vi "Set MAX Volts.vi"(8 "error in (no error)":errorcluster, 11 "VISA resource name":refnum<visa-resource-name>) -> (0 "error out":errorcluster, 3 "VISA resource name out":refnum<visa-resource-name>)   [LabVIEW 2010, in "Agilent U2722.lvlib"]
doc: "Configures the channel to output in source voltage mode."
uses:
  U2722 LabVIEW Instr Driver and Examples/Agilent U2722.lvlib
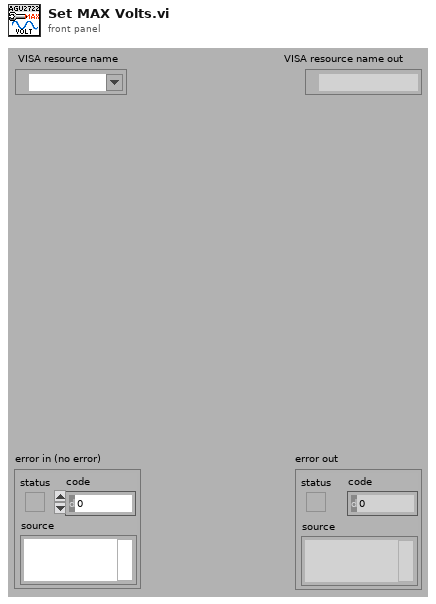
[diagram p1: front panel]
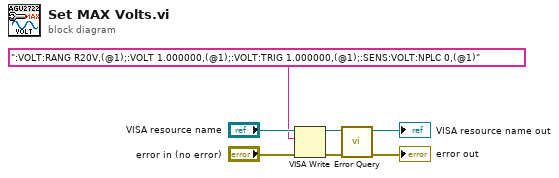
[diagram p0: block diagram]
diagram:
  n1 = VISA Write(VISA resource name="VISA resource name", write buffer=":VOLT:RANG R20V,(@1);:VOLT 1.000000,(@1);:VOLT:TRIG 1.000000,(@1);:SENS:VOLT:NPLC 0,(@1)" ("resulting string"), error in (no error)="error in (no error)") -> (VISA resource name out=w3:refnum<visa-resource-name>, error out=w2:errorcluster)  [unwired: 1 out]
  n2 = call "Error Query.vi"("error in (no error)"=w2, "VISA resource name"=w3) -> ("error out"=→"error out":errorcluster, "VISA resource name out"=→"VISA resource name out":refnum<visa-resource-name>)  [unwired: 6 in, 2 out]
